vi "CH_LM DFM Create Directory.vi"(0 "Meter Index":i32, 2 "Directory Name (\"\")":string, 5 "error in (no error)":errorcluster, 7 "Timeout / ms (3000)":i32=3000, 9 "Lock Timeout / ms (1000)":i32=1000) -> (11 "Lock timed out":bool, 14 "Meter Index":i32, 19 "error out":errorcluster)   [LabVIEW 2012, in "CH_LM.lvlib"]
doc: "This command will create a new directory.\n\n<B>Attention:</B> An attempt to create an existing directory will raise error 202. An attempt to create a directory using the name of an existing file will raise error 202. An attempt to create a new directory when the storage volume is full will raise error -254."
uses:
  CH_LM.lvlib
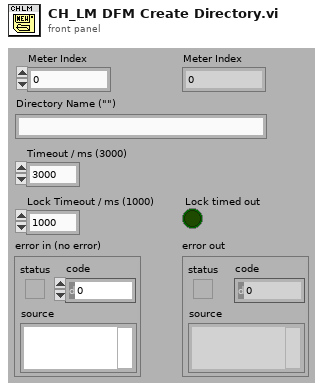
[diagram p1: front panel]
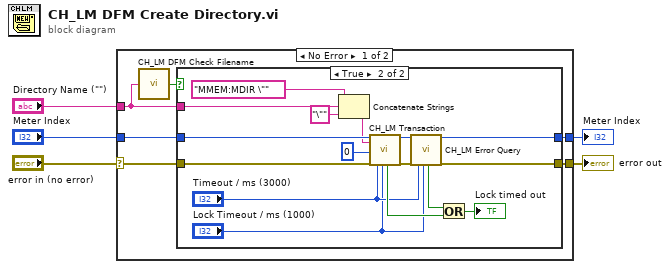
[diagram p0: block diagram]
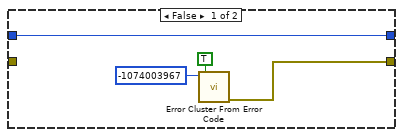
[diagram p2: hidden frame]
diagram:
  n1 = case shown="No Error" "error in (no error)" {
    selector: "error in (no error)" -> [w11 w33]
    tunnel: [w8 w33] -> w5
    tunnel: "Meter Index" -> [w10 w32]
    tunnel: [w9 w32] -> w2
    tunnel: "Directory Name (\"\")" -> [w7 _]
    frame No Error {
      n2 = call "CH_LM DFM Check Filename.vi"("Directory or File Name (\"\")"=w7) -> ("Valid"=w6:bool)
      n3 = case shown="True" w6 {
        tunnel: w11 -> [_ w31]
        tunnel: w10 -> [w15 w30]
        tunnel: [w15 w29] -> w9
        tunnel: [w12 w28] -> w8
        tunnel: w7 -> [_ w27]
        frame False {
          n4 = call <vilib>:"Error Cluster From Error Code.vi"("show call chain? (False)"=TRUE, "error code (0)"=-1074003967) -> ("error out"=w12:errorcluster)  [unwired: 1 in, 6 out]
        }
        frame True {
          n5 = Concatenate Strings("MMEM:MDIR \"" ("Command String"), w27, "\"" ("string")) -> (w18:string)
          n6 = call "CH_LM Transaction.vi"("Meter Index"=w30, "Command String"=w18, "NofStrings (-1:all)"=0 ("t"), "error in (no error)"=w31, "Timeout / ms (3000)"="Timeout / ms (3000)", "Lock Timeout / ms (1000)"="Lock Timeout / ms (1000)") -> ("Lock timed out"=w22:bool, "Meter Index"=w25:i32, "error out"=w24:errorcluster)  [unwired: 11 out]
          n7 = call "CH_LM Error Query.vi"("Meter Index"=w25, "error in (no error)"=w24, "Timeout / ms (3000)"="Timeout / ms (3000)", "Lock Timeout / ms (1000)"="Lock Timeout / ms (1000)") -> ("Lock timed out"=w23:bool, "Meter Index"=w29:i32, "error out"=w28:errorcluster)  [unwired: 13 out]
          n8 = Or(x=w23, y=w22) -> (x .or. y?=→"Lock timed out":bool)
        }
      }
    }
    frame Error {
    }
  }
  "error out" <- w5
  "Meter Index" <- w2
